vi "CRYGet Freq From Flatten Data.vi"(10 "Flattened Element Data":string, 11 "Stimulus Type":string) -> (2 "Stop Freq(Hz)":dbl, 3 "Start Freq(Hz)":dbl)   [LabVIEW 2013]
uses:
  Control/CRYfstepsw.ctl
  Control/CRYflogsw.ctl
  Control/CRYtwotone.ctl
  Control/CRYnoise.ctl
  Control/CRYmltitone.ctl
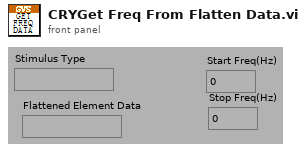
[diagram p1: front panel]
types:
  T1 = typedef "CRYfstepsw.ctl" = cluster{"Level(U)":dbl, "Start Freq(Hz)":dbl, "Stop Freq(Hz)":dbl, "ML val level name":string, "Use ML Val level?":bool, "ML axis":u8, "Steps (#)":i32, "Cycles/step(#)":u32, "Time/step (s)":dbl, "Step Resolution":u16, "unit":u16, "Start Freq Name":string, "Stop Freq Name":string, "Start Freq Axis":u8, "Stop Freq Axis":u8, "Start Freq Flag":string, "Stop Freq Flag":string, "Output Imp":dbl, "Nominal Imp":dbl, "V on DUT":bool}
  T2 = typedef "CRYflogsw.ctl" = cluster{"Level(U)":dbl, "Start Freq(Hz)":dbl, "Stop Freq(Hz)":dbl, "Sweep Rate(s/dec)":dbl, "Use ML Val level?":bool, "ML val level name":string, "ML axis":u8, "TSR params":cluster{"FSamp":dbl, "FStart":dbl, "FStop":dbl, "NOffset":dbl, "MStop":dbl, "MStart":dbl, "NHarm":dbl, "Tsamp":dbl, "Amplit":dbl}, "unit":u16, "Start Freq Name":string, "Stop Freq Name":string, "Start Freq Axis":u8, "Stop Freq Axis":u8, "Start Freq Flag":string, "Stop Freq Flag":string, "Output Imp":dbl, "Nominal Imp":dbl, "V on DUT":bool}
  T3 = typedef "CRYtwotone.ctl" = cluster{"Steps (#)":i32, "Tone Type":u8, "Freq2(Hz)":dbl, "Time/step (s)":dbl, "Cycles/step (#)":u32, "ML val level name":string, "Use ML Val level?":bool, "Level(U) 2":dbl, "Diff Freq(Hz)":dbl, "ML axis 2":u8, "Diff/Ratio":u8, "Level(U)":dbl, "Stop Freq(Hz)":dbl, "Ratio Val":dbl, "ML val level name 2":string, "Use ML Val level? 2":bool, "ML axis":u8, "Start Freq(Hz)":dbl, "Step Resolution":u16, "Ratio":u16, "TabCtrl6":enum32{"Master Tone", "Slave Tone"}, "unit 1":u16, "unit 2":u16, "Start Freq Name":string, "Stop Freq Name":string, "Start Freq Axis":u8, "Stop Freq Axis":u8, "Start Freq Flag":string, "Stop Freq Flag":string}
  T4 = typedef "CRYnoise.ctl" = cluster{"Noise Type":u8, "Min Freq(Hz)":dbl, "Max Freq(Hz)":dbl, "Level(U)":dbl, "Duration(s)":dbl, "ML val level name":string, "Use ML Val level?":bool, "ML axis":u8, "unit":u16, "Start Freq Name":string, "Stop Freq Name":string, "Start Freq Axis":u8, "Stop Freq Axis":u8, "Start Freq Flag":string, "Stop Freq Flag":string, "Output Imp":dbl, "Nominal Imp":dbl, "V on DUT":bool}
  T5 = typedef "CRYmltitone.ctl" = cluster{"Level(U)":dbl, "Min Freq(Hz)":dbl, "Max Freq(Hz)":dbl, "Duration(s)":dbl, "Freq Rounding":bool, "Rounding Val":dbl, "Profile":i32, "ML axis 2":u8, "ML val level name":string, "Use ML Val level?":bool, "ML axis":u8, "Step Resolution":u16, "unit":u16, "Start Freq Name":string, "Stop Freq Name":string, "Start Freq Axis":u8, "Stop Freq Axis":u8, "Start Freq Flag":string, "Stop Freq Flag":string, "Output Imp":dbl, "Nominal Imp":dbl, "V on DUT":bool}
  T6 = typedef "CRYData Cluster.ctl" = cluster{"Name":string, "Curve":cluster{"x":dbl, "y":dbl, "z":dbl}[], "X data":u16, "Y data":u16, "Z data":u16, "X axis":u16, "Y axis":u16, "Z axis":u16, "X unit":string, "Y unit":string, "Z unit":string, "X dB ref":dbl, "Y dB ref":dbl, "Z dB ref":dbl, "single val":bool, "protected":bool, "display X":bool, "display Y":bool, "display Z":bool, "Test Info":string, "Step No.":i32, "Plot Settings":cluster{"Color":u32, "Interpolation":u8, "Point Style":u8, "Line Style":u8, "Point Color":u32, "Line Width":u8, "Bar Plot Style":u8, "Fill To":i16}, "AutoProtect":bool}
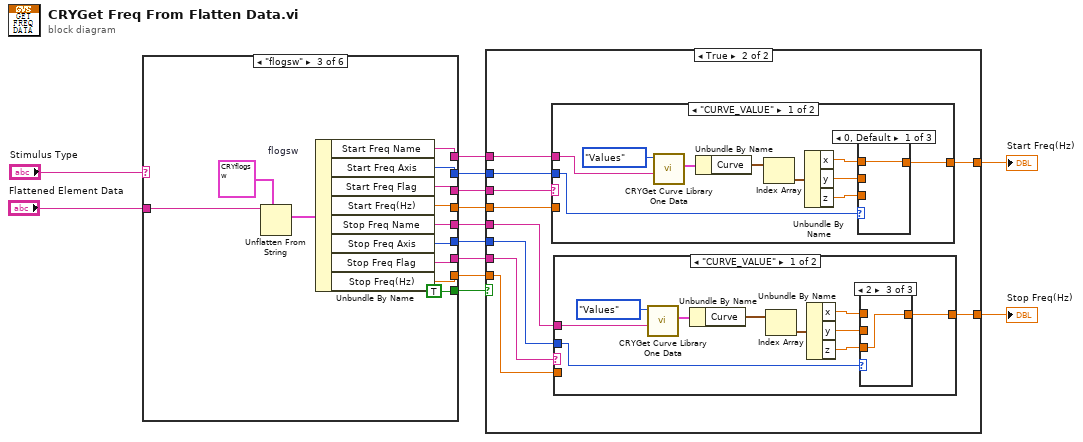
[diagram p0: block diagram]
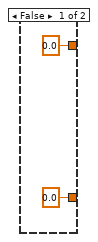
[diagram p2: hidden frame]
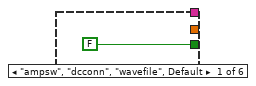
[diagram p9: hidden frame]
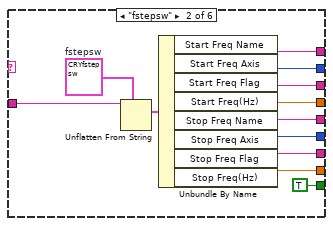
[diagram p10: hidden frame]
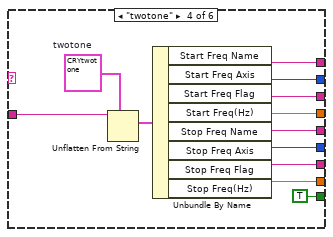
[diagram p11: hidden frame]
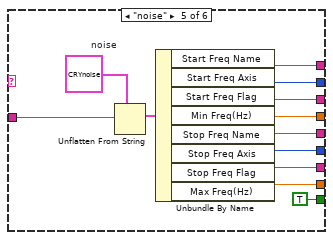
[diagram p12: hidden frame]
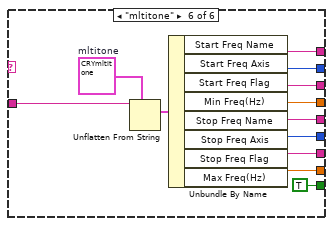
[diagram p13: hidden frame]
diagram:
  n1 = case shown="\"flogsw\"" "Stimulus Type" {
    tunnel: "Flattened Element Data" -> [_ w26 w38 w50 w62 w74]
    tunnel: [_ w23 w35 w47 w59 w71] -> w8
    tunnel: [_ w22 w34 w46 w58 w70] -> w7
    tunnel: [_ w21 w33 w45 w57 w69] -> w6
    tunnel: [_ w20 w32 w44 w56 w68] -> w5
    tunnel: [_ w19 w31 w43 w55 w67] -> w4
    tunnel: [_ w18 w30 w42 w54 w66] -> w3
    tunnel: [_ w17 w29 w41 w53 w65] -> w2
    tunnel: [_ w16 w28 w40 w52 w64] -> w1
    tunnel: [FALSE TRUE TRUE TRUE TRUE TRUE] -> w9
    frame "ampsw", "dcconn", "wavefile", Default {
    }
    frame "fstepsw" {
      w24 = T1 {"Level(U)"=0.7071067811865476, "Start Freq(Hz)"=20000.0, "Stop Freq(Hz)"=20.0, "ML val level name"="Calibration sens-out Left", "Use ML Val level?"=FALSE, "ML axis"=0, "Steps (#)"=31, "Cycles/step(#)"=20, "Time/step (s)"=0.01, "Step Resolution"=0, "unit"=0, "Start Freq Name"="Calibration sens-out Left", "Stop Freq Name"="Calibration sens-out Left", "Start Freq Axis"=0, "Stop Freq Axis"=0, "Start Freq Flag"="", "Stop Freq Flag"="", "Output Imp"=0.0, "Nominal Imp"=0.0, "V on DUT"=FALSE}  # fstepsw
      n2 = Unflatten From String(type=w24, binary string=w26) -> (value=w25:T1)  [unwired: 1 in, 4 out]
      n3 = Unbundle By Name(w25) -> ("Start Freq Name"=w23:string, "Start Freq Axis"=w22:u8, "Start Freq Flag"=w21:string, "Start Freq(Hz)"=w20:dbl, "Stop Freq Name"=w19:string, "Stop Freq Axis"=w18:u8, "Stop Freq Flag"=w17:string, "Stop Freq(Hz)"=w16:dbl)
    }
    frame "flogsw" {
      w37 = T2 {"Level(U)"=1.0, "Start Freq(Hz)"=100.0, "Stop Freq(Hz)"=6300.0, "Sweep Rate(s/dec)"=1.0, "Use ML Val level?"=FALSE, "ML val level name"="", "ML axis"=1, "TSR params"={"FSamp"=0.0, "FStart"=0.0, "FStop"=0.0, "NOffset"=0.0, "MStop"=0.0, "MStart"=0.0, "NHarm"=0.0, "Tsamp"=0.0, "Amplit"=0.0}, "unit"=0, "Start Freq Name"="Calibration sens-out Left", "Stop Freq Name"="Calibration sens-out Left", "Start Freq Axis"=0, "Stop Freq Axis"=0, "Start Freq Flag"="", "Stop Freq Flag"="", "Output Imp"=0.0, "Nominal Imp"=0.0, "V on DUT"=FALSE}  # flogsw
      n4 = Unflatten From String(type=w37, binary string=w38) -> (value=w36:T2)  [unwired: 1 in, 4 out]
      n5 = Unbundle By Name(w36) -> ("Start Freq Name"=w35:string, "Start Freq Axis"=w34:u8, "Start Freq Flag"=w33:string, "Start Freq(Hz)"=w32:dbl, "Stop Freq Name"=w31:string, "Stop Freq Axis"=w30:u8, "Stop Freq Flag"=w29:string, "Stop Freq(Hz)"=w28:dbl)
    }
    frame "twotone" {
      w49 = T3 {"Steps (#)"=19, "Tone Type"=0, "Freq2(Hz)"=1000.0, "Time/step (s)"=0.0, "Cycles/step (#)"=12, "ML val level name"="", "Use ML Val level?"=FALSE, "Level(U) 2"=1.0, "Diff Freq(Hz)"=100.0, "ML axis 2"=1, "Diff/Ratio"=0, "Level(U)"=1.0, "Stop Freq(Hz)"=100.0, "Ratio Val"=0.8, "ML val level name 2"="", "Use ML Val level? 2"=FALSE, "ML axis"=1, "Start Freq(Hz)"=6300.0, "Step Resolution"=0, "Ratio"=0, "TabCtrl6"=enum."Master Tone", "unit 1"=0, "unit 2"=0, "Start Freq Name"="", "Stop Freq Name"="", "Start Freq Axis"=0, "Stop Freq Axis"=0, "Start Freq Flag"="", "Stop Freq Flag"=""}  # twotone
      n6 = Unflatten From String(type=w49, binary string=w50) -> (value=w48:T3)  [unwired: 1 in, 4 out]
      n7 = Unbundle By Name(w48) -> ("Start Freq Name"=w47:string, "Start Freq Axis"=w46:u8, "Start Freq Flag"=w45:string, "Start Freq(Hz)"=w44:dbl, "Stop Freq Name"=w43:string, "Stop Freq Axis"=w42:u8, "Stop Freq Flag"=w41:string, "Stop Freq(Hz)"=w40:dbl)
    }
    frame "noise" {
      w61 = T4 {"Noise Type"=0, "Min Freq(Hz)"=20.0, "Max Freq(Hz)"=20000.0, "Level(U)"=1.0, "Duration(s)"=1.0, "ML val level name"="", "Use ML Val level?"=FALSE, "ML axis"=1, "unit"=0, "Start Freq Name"="", "Stop Freq Name"="", "Start Freq Axis"=0, "Stop Freq Axis"=0, "Start Freq Flag"="", "Stop Freq Flag"="", "Output Imp"=0.0, "Nominal Imp"=0.0, "V on DUT"=FALSE}  # noise
      n8 = Unflatten From String(type=w61, binary string=w62) -> (value=w60:T4)  [unwired: 1 in, 4 out]
      n9 = Unbundle By Name(w60) -> ("Start Freq Name"=w59:string, "Start Freq Axis"=w58:u8, "Start Freq Flag"=w57:string, "Min Freq(Hz)"=w56:dbl, "Stop Freq Name"=w55:string, "Stop Freq Axis"=w54:u8, "Stop Freq Flag"=w53:string, "Max Freq(Hz)"=w52:dbl)
    }
    frame "mltitone" {
      w73 = T5 {"Level(U)"=0.0, "Min Freq(Hz)"=0.0, "Max Freq(Hz)"=0.0, "Duration(s)"=0.0, "Freq Rounding"=FALSE, "Rounding Val"=5.0, "Profile"=0, "ML axis 2"=0, "ML val level name"="", "Use ML Val level?"=FALSE, "ML axis"=0, "Step Resolution"=0, "unit"=0, "Start Freq Name"="Calibration sens-out Left", "Stop Freq Name"="Calibration sens-out Left", "Start Freq Axis"=0, "Stop Freq Axis"=0, "Start Freq Flag"="", "Stop Freq Flag"="", "Output Imp"=0.0, "Nominal Imp"=0.0, "V on DUT"=FALSE}  # mltitone
      n10 = Unflatten From String(type=w73, binary string=w74) -> (value=w72:T5)  [unwired: 1 in, 4 out]
      n11 = Unbundle By Name(w72) -> ("Start Freq Name"=w71:string, "Start Freq Axis"=w70:u8, "Start Freq Flag"=w69:string, "Min Freq(Hz)"=w68:dbl, "Stop Freq Name"=w67:string, "Stop Freq Axis"=w66:u8, "Stop Freq Flag"=w65:string, "Max Freq(Hz)"=w64:dbl)
    }
  }
  n12 = case shown="True" w9 {
    tunnel: [0.0 ("Min Freq(Hz)") w86] -> w11
    tunnel: [0.0 ("Max Freq(Hz)") w85] -> w10
    tunnel: w8 -> [_ w84]
    tunnel: w7 -> [_ w83]
    tunnel: w6 -> [_ w82]
    tunnel: w5 -> [_ w81]
    tunnel: w4 -> [_ w80]
    tunnel: w3 -> [_ w77]
    tunnel: w2 -> [_ w79]
    tunnel: w1 -> [_ w78]
    frame False {
    }
    frame True {
      n13 = case shown="\"CURVE_VALUE\"" w82 {
        tunnel: [w105 w114] -> w86
        tunnel: w84 -> [w102 _]
        tunnel: w83 -> [w101 _]
        tunnel: w81 -> [_ w114]
        frame "CURVE_VALUE" {
          n14 = call "CRYGet Curve Library One Data .vi"("Data Name"=w102, "Type"=enum16{"Curves", "Values", "Results", "WFM"}."Values") -> ("Value"=w109:T6)  [unwired: 3 in, 6 out]
          n15 = Unbundle By Name(w109) -> ("Curve"=w108:cluster{"x":dbl, "y":dbl, "z":dbl}[])
          n16 = Index Array(array=w108) -> (element=w107:cluster{"x":dbl, "y":dbl, "z":dbl})  [unwired: 1 in]
          n17 = Unbundle By Name(w107) -> ("x"=w106:dbl, "y"=w104:dbl, "z"=w103:dbl)
          n18 = case shown="0, Default" w101 {
            tunnel: [w111 w112 w113] -> w105
            tunnel: w106 -> [w111 _ _]
            tunnel: w104 -> [_ w112 _]
            tunnel: w103 -> [_ _ w113]
            frame 0, Default {
            }
            frame 1 {
            }
            frame 2 {
            }
          }
        }
        frame "USER_INPUT", Default {
        }
      }
      n19 = case shown="\"CURVE_VALUE\"" w79 {
        tunnel: [w91 w100] -> w85
        tunnel: w80 -> [w88 _]
        tunnel: w78 -> [_ w100]
        tunnel: w77 -> [w87 _]
        frame "CURVE_VALUE" {
          n20 = call "CRYGet Curve Library One Data .vi"("Data Name"=w88, "Type"=enum16{"Curves", "Values", "Results", "WFM"}."Values") -> ("Value"=w95:T6)  [unwired: 3 in, 6 out]
          n21 = Unbundle By Name(w95) -> ("Curve"=w94:cluster{"x":dbl, "y":dbl, "z":dbl}[])
          n22 = Index Array(array=w94) -> (element=w93:cluster{"x":dbl, "y":dbl, "z":dbl})  [unwired: 1 in]
          n23 = Unbundle By Name(w93) -> ("x"=w92:dbl, "y"=w90:dbl, "z"=w89:dbl)
          n24 = case shown="2" w87 {
            tunnel: [w97 w98 w99] -> w91
            tunnel: w92 -> [w97 _ _]
            tunnel: w90 -> [_ w98 _]
            tunnel: w89 -> [_ _ w99]
            frame 0, Default {
            }
            frame 1 {
            }
            frame 2 {
            }
          }
        }
        frame "USER_INPUT", Default {
        }
      }
    }
  }
  "Start Freq(Hz)" <- w11
  "Stop Freq(Hz)" <- w10
